vi "ADC Command.vi"(0 "Serial Device in":refnum<class "Serial Device.lvclass">, 1 "Serial Device Brand":string, 11 "error in (no error)":errorcluster) -> (4 "Serial Device out":refnum<class "Serial Device.lvclass">, 6 "Command to send":string, 8 "Expected Command":string, 15 "error out":errorcluster)   [LabVIEW 2020, in "Serial Device.lvclass"]
uses:
  Serial Device.lvclass
panel:
  in  "Channel":u8
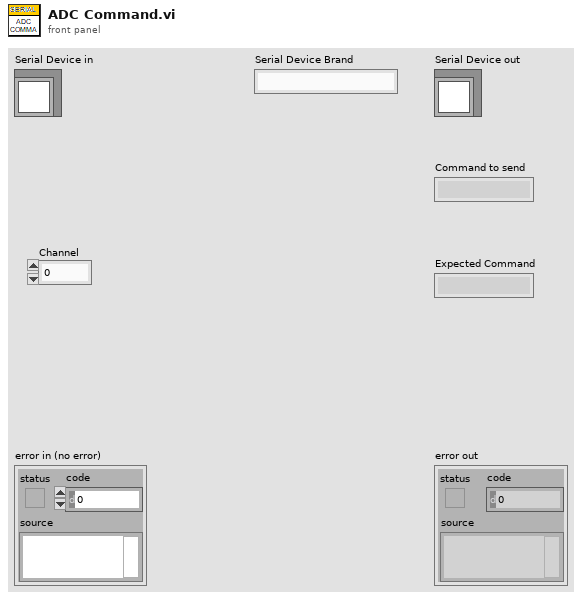
[diagram p1: front panel]
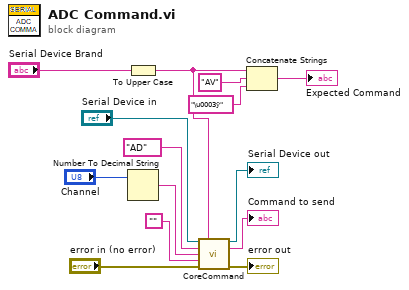
[diagram p0: block diagram]
diagram:
  n1 = To Upper Case(1:"Serial Device Brand") -> (0:w3:string)
  n2 = Number To Decimal String(number="Channel") -> (decimal integer string=w5:string)  [unwired: 1 in]
  n3 = call-dynamic "CoreCommand.vi"("Serial Device in"="Serial Device in", "Serial Device Brand"=w3, "Command"="AD", "Param 1"=w5, "Param 2"="", "error in (no error)"="error in (no error)") -> ("Serial Device out"=→"Serial Device out":refnum<class "Serial Device.lvclass">, "Command to send"=→"Command to send":string, "error out"=→"error out":errorcluster)  [unwired: 6 in, 1 out]
  n4 = Concatenate Strings(w3, "AV" ("string"), "\u0003ÿ" ("string")) -> (→"Expected Command":string)
